vi "Element Type.vi"(11 "LocalGraphBuffer in":refnum<class "LocalGraphBuffer.lvclass">) -> (2 "Element Type":string)   [LabVIEW 2020, in "VolatusGUIElements.lvlib" / "LocalGraphBuffer.lvclass"]
uses:
  LocalGraphBuffer.lvclass
  LocalGraphBuffer.lvclass/LocalGraphBuffer.ctl
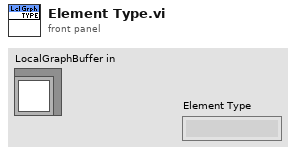
[diagram p1: front panel]
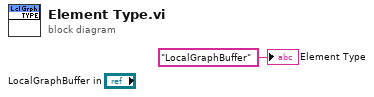
[diagram p0: block diagram]
diagram:
  "Element Type" <- "LocalGraphBuffer" ("Element Type")
